vi "ADI_IMU_ADIS16448_Close.vi"(8 "error in":errorcluster, 11 "ADI IMU DevRef":T1={"DevStatus"={"status"=FALSE, "code"=0, "source"=""}, "Handle"=27, "SPI Bus"=enum."SPI MXP", "Device Found"=TRUE, "Device Ready"=FALSE, "Yaw Axis"=enum."Z", "AHRS Algorithm"=enum."Complementary", "Serial"=118, "Lot ID 2"=5379, "Lot ID 1"=118, "Bytes Per Sample"=0, "Calibrate On Open?"=FALSE}) -> (0 "error out":errorcluster)   [LabVIEW 2017, in "ADIS16448_IMU.lvlib"]
doc: "Closes the ADIIMUDevRef and properly shuts down SPI communication between the RoboRIO and the ADI IMU MXP board."
uses:
  Desktop/ADIS16448/ADIS16448-RoboRIO-Driver-master/LabVIEW/ADIS16448 IMU/ADIS16448_IMU.lvlib
  Desktop/ADIS16448/ADIS16448-RoboRIO-Driver-master/LabVIEW/ADIS16448 IMU/ADI_IMU_ADIS16448_IMUDevRef.ctl
  <vilib>/Rock Robotics/SystemInterfaces/spilib/spi_bus.ctl
  <vilib>/Rock Robotics/WPI/SPI/WPI_SPIDevRef.ctl
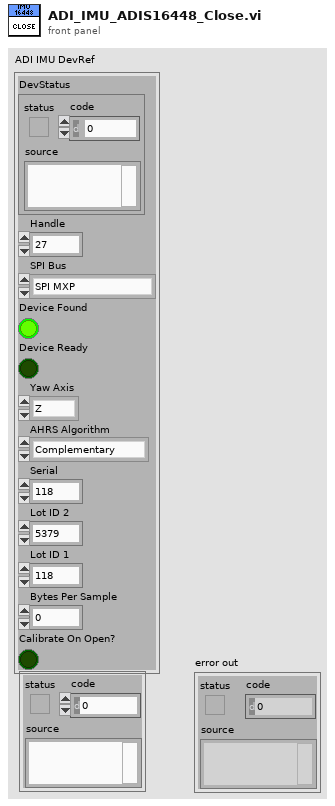
[diagram p1: front panel]
types:
  T1 = typedef "ADIS16448_IMU.lvlib/ADI_IMU_ADIS16448_IMUDevRef.ctl" = cluster{"DevStatus":errorcluster, "Handle":i32, "SPI Bus":T2, "Device Found":bool, "Device Ready":bool, "Yaw Axis":enum16{"X", "Y", "Z"}, "AHRS Algorithm":enum16{"Complementary", "Madgwick"}, "Serial":u16, "Lot ID 2":u16, "Lot ID 1":u16, "Bytes Per Sample":u16, "Calibrate On Open?":bool}
  T2 = typedef "spi_bus.ctl" = enum16{"SPI On-Board, CS0", "SPI On-Board, CS1", "SPI On-Board, CS2", "SPI On-Board, CS3", "SPI MXP", "Invalid"}
  T3 = typedef "WPI_SPIDevRef.ctl" = cluster{"DevStatus":errorcluster, "Handle":i32, "SPI Bus":T2}
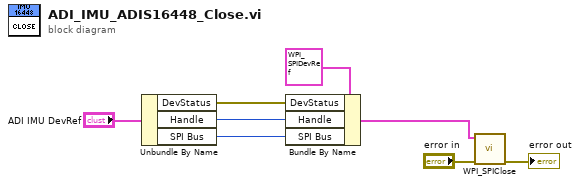
[diagram p0: block diagram]
diagram:
  n1 = Unbundle By Name("ADI IMU DevRef") -> ("DevStatus"=w4:errorcluster, "Handle"=w3:i32, "SPI Bus"=w2:T2)
  n2 = Bundle By Name(cluster=T3 {"DevStatus"={"status"=FALSE, "code"=0, "source"=""}, "Handle"=0, "SPI Bus"=enum."SPI On-Board, CS0"} ("SPIDevRef"), "DevStatus"=w4, "Handle"=w3, "SPI Bus"=w2) -> (w6:T3)
  n3 = call <vilib>:"WPI_SPIClose.vi"("error in (no error)"="error in", "SPIDevRef"=w6) -> ("error out"=→"error out":errorcluster)  [unwired: 9 in]
